vi "main.vi"() -> ()   [LabVIEW 2016]
uses:
  SALLV_Test/DataTypes/ackcmd.ctl
  SALLV_Test/DataTypes/logevent_arrays.ctl
  SALLV_Test/DataTypes/arrays.ctl
  SALLV_Test/DataTypes/logevent_scalars.ctl
  SALLV_Test/DataTypes/scalars.ctl
  SALLV_Test/VIs/Test_logEvent_summaryState.vi
  SALLV_Test/SALLV_Test.lvlib
panel:
  in  "TestID":u32
  out "Stop":bool
  in  "SummaryState":i32=5
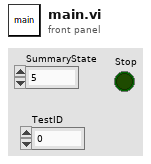
[diagram p1: front panel]
types:
  T1 = typedef "SALLV_Test.lvlib/ackcmd.ctl" = cluster{"cmdSeqNum":i32, "ack":i32, "error":i32, "result":string}
  T2 = typedef "SALLV_Test.lvlib/arrays.ctl" = cluster{"boolean0[5]":bool[], "byte0[5]":u8[], "char0":string, "short0[5]":i16[], "int0[5]":i32[], "long0[5]":i32[], "longLong0[5]":i64[], "octet0[5]":u8[], "unsignedShort0[5]":u16[], "unsignedInt0[5]":u32[], "unsignedLong0[5]":u32[], "float0[5]":sgl[], "double0[5]":dbl[]}
  T3 = typedef "SALLV_Test.lvlib/logevent_arrays.ctl" = cluster{"boolean0[5]":bool[], "byte0[5]":u8[], "char0":string, "short0[5]":i16[], "int0[5]":i32[], "long0[5]":i32[], "longLong0[5]":i64[], "octet0[5]":u8[], "unsignedShort0[5]":u16[], "unsignedInt0[5]":u32[], "unsignedLong0[5]":u32[], "float0[5]":sgl[], "double0[5]":dbl[], "priority":i32}
  T4 = typedef "SALLV_Test.lvlib/scalars.ctl" = cluster{"boolean0":bool, "byte0":u8, "char0":string, "short0":i16, "int0":i32, "long0":i32, "longLong0":i64, "octet0":u8, "unsignedShort0":u16, "unsignedInt0":u32, "unsignedLong0":u32, "float0":sgl, "double0":dbl, "string0":string}
  T5 = typedef "SALLV_Test.lvlib/logevent_scalars.ctl" = cluster{"boolean0":bool, "byte0":u8, "char0":string, "short0":i16, "int0":i32, "long0":i32, "longLong0":i64, "octet0":u8, "unsignedShort0":u16, "unsignedInt0":u32, "unsignedLong0":u32, "float0":sgl, "double0":dbl, "string0":string, "priority":i32}
  T6 = typedef "SALLV_Test.lvlib/command_setArrays.ctl" = cluster{"boolean0[5]":bool[], "byte0[5]":u8[], "char0":string, "short0[5]":i16[], "int0[5]":i32[], "long0[5]":i32[], "longLong0[5]":i64[], "octet0[5]":u8[], "unsignedShort0[5]":u16[], "unsignedInt0[5]":u32[], "unsignedLong0[5]":u32[], "float0[5]":sgl[], "double0[5]":dbl[]}
  T7 = typedef "SALLV_Test.lvlib/command_setScalars.ctl" = cluster{"boolean0":bool, "byte0":u8, "char0":string, "short0":i16, "int0":i32, "long0":i32, "longLong0":i64, "octet0":u8, "unsignedShort0":u16, "unsignedInt0":u32, "unsignedLong0":u32, "float0":sgl, "double0":dbl, "string0":string}
  T8 = typedef "SALLV_Test.lvlib/command_wait.ctl" = cluster{"cmdSeqNum":i32, "ack":i32, "duration":dbl}
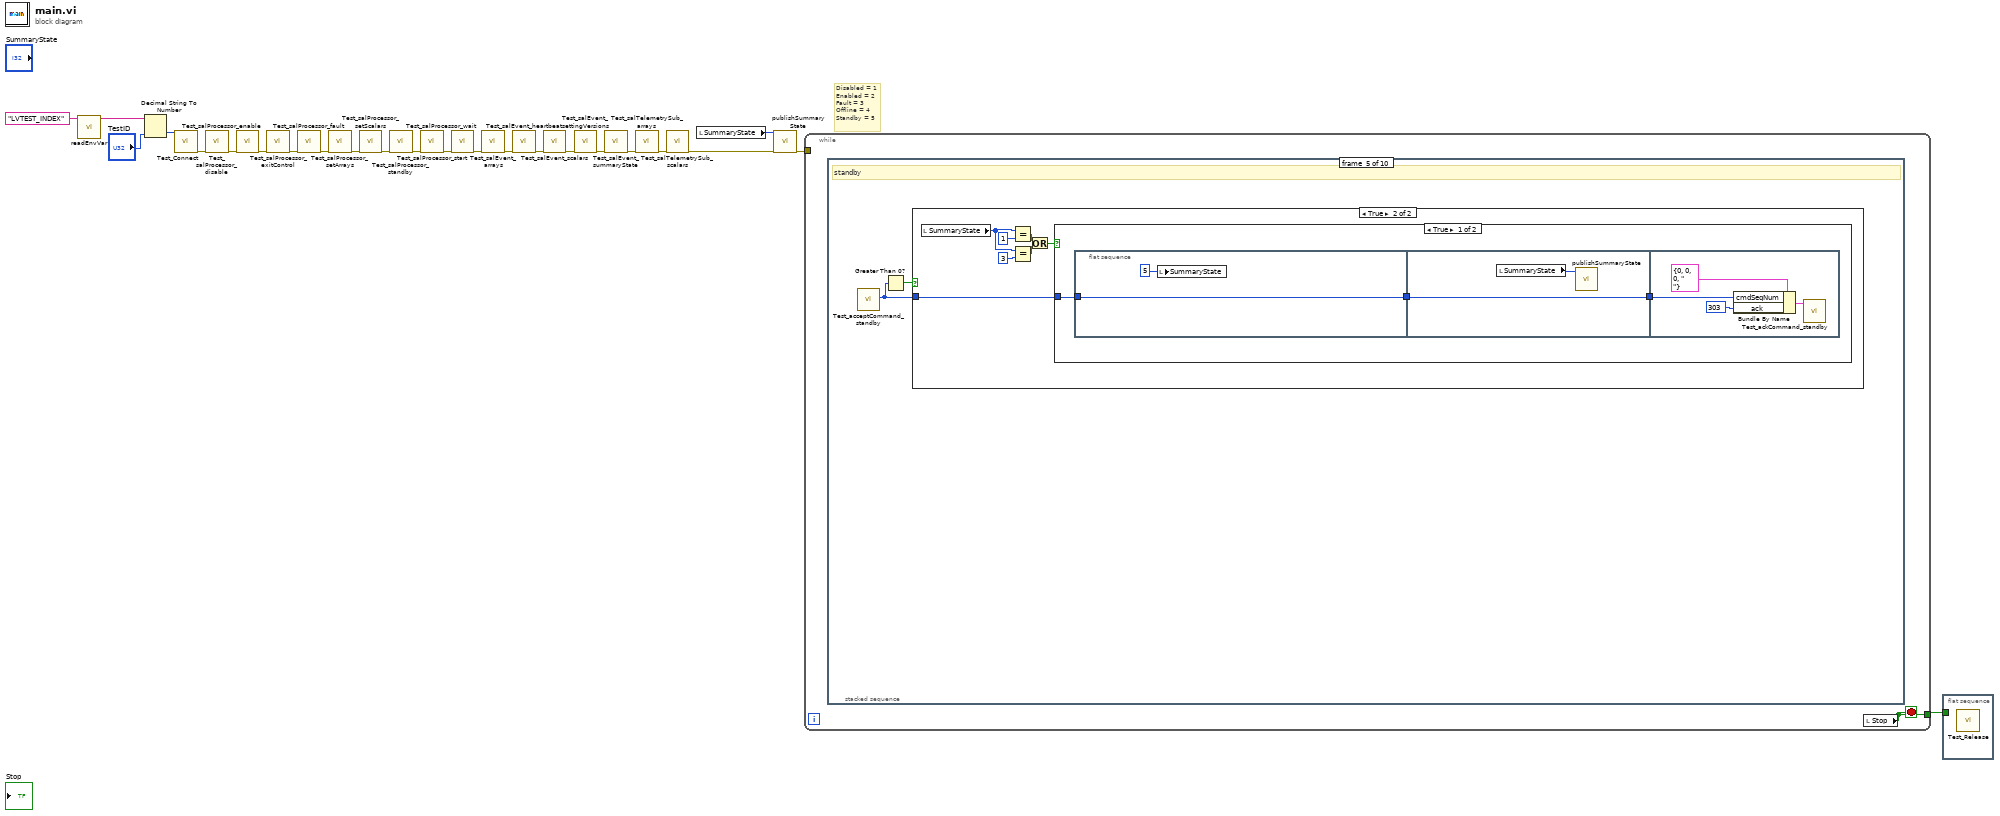
[diagram p0: block diagram]
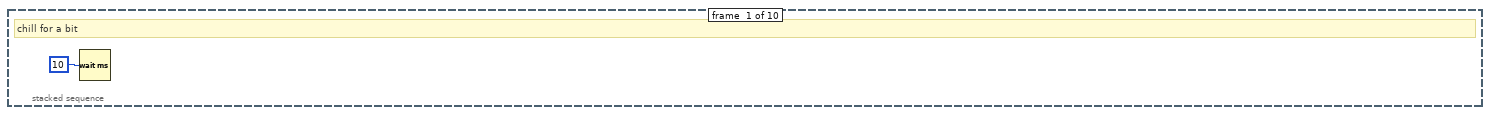
[diagram p2: hidden frame]
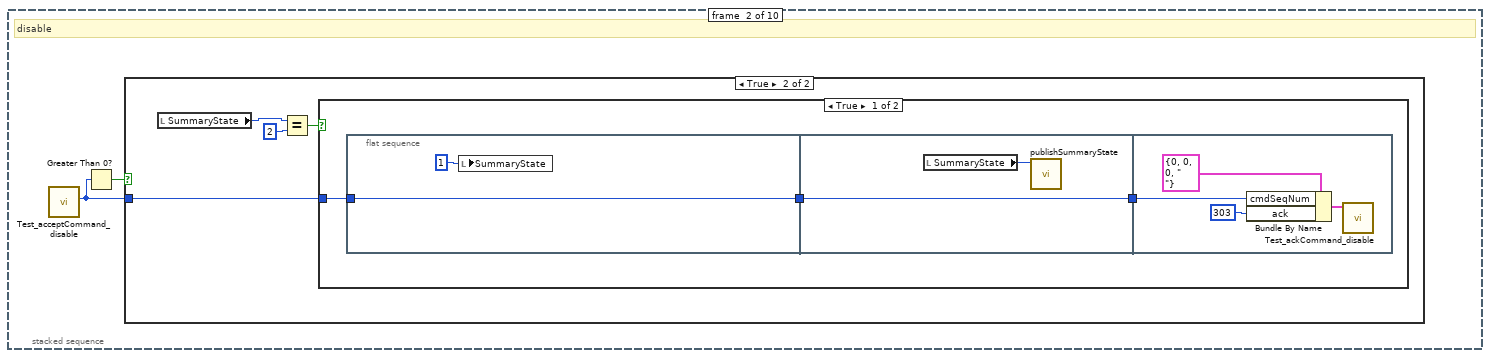
[diagram p3: hidden frame]
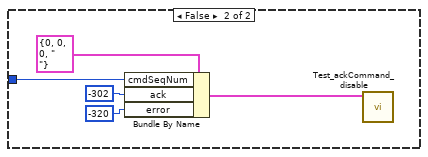
[diagram p5: hidden frame]
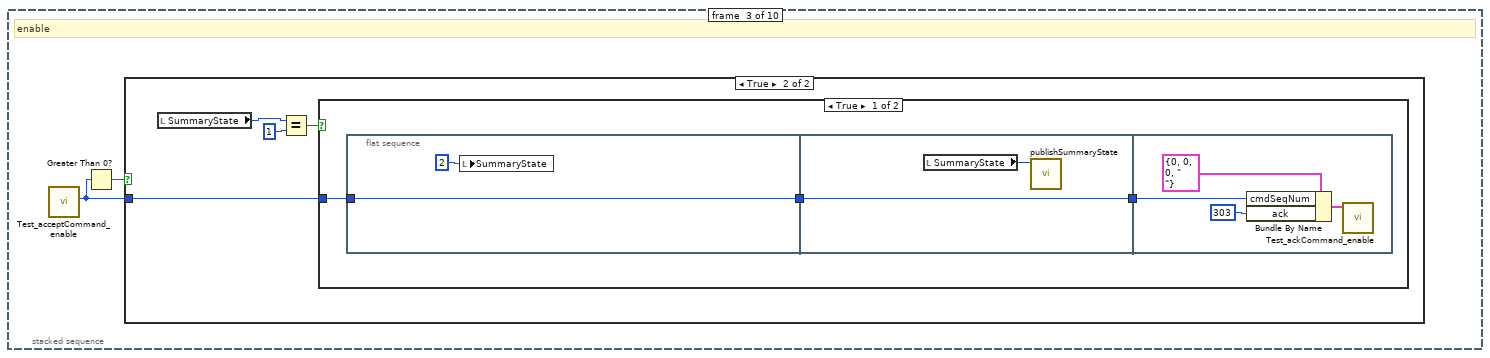
[diagram p6: hidden frame]
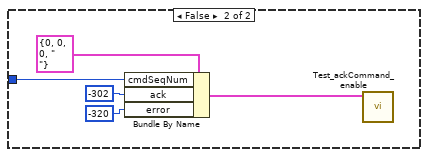
[diagram p8: hidden frame]
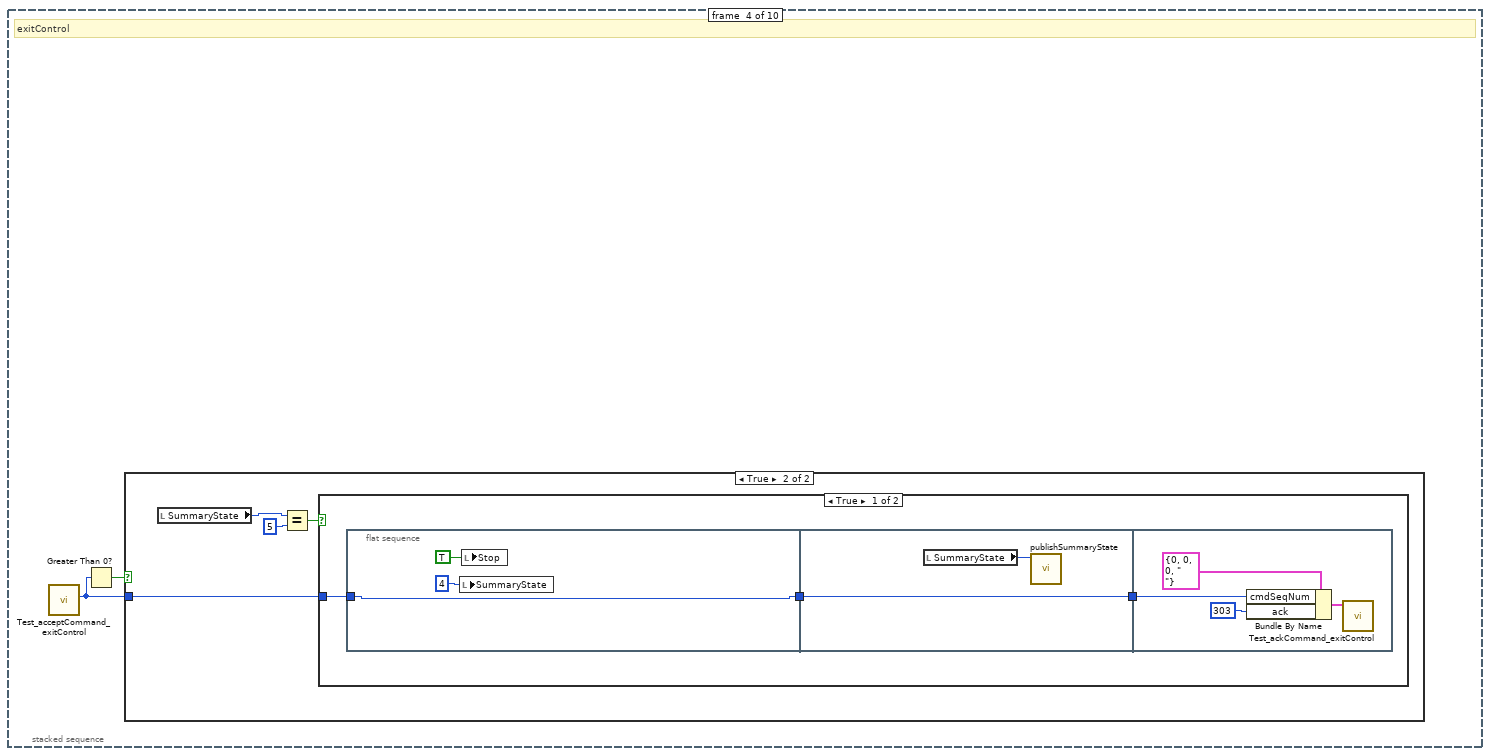
[diagram p9: hidden frame]
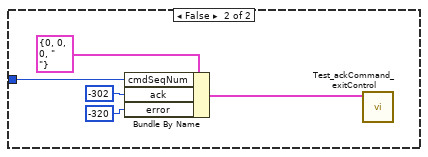
[diagram p11: hidden frame]
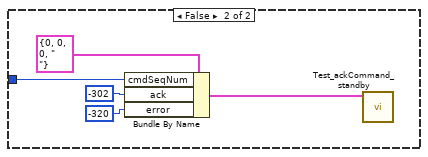
[diagram p13: hidden frame]
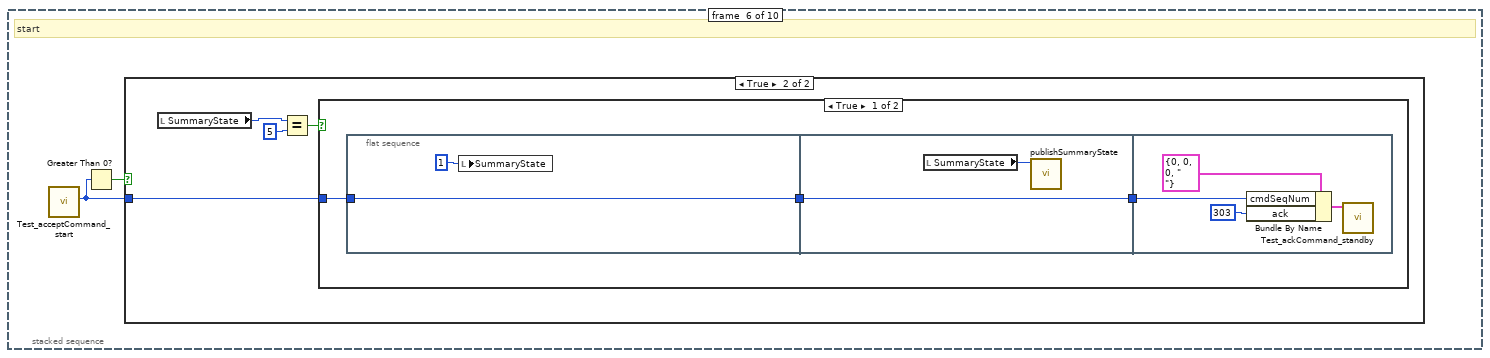
[diagram p14: hidden frame]
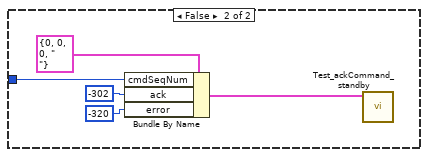
[diagram p16: hidden frame]
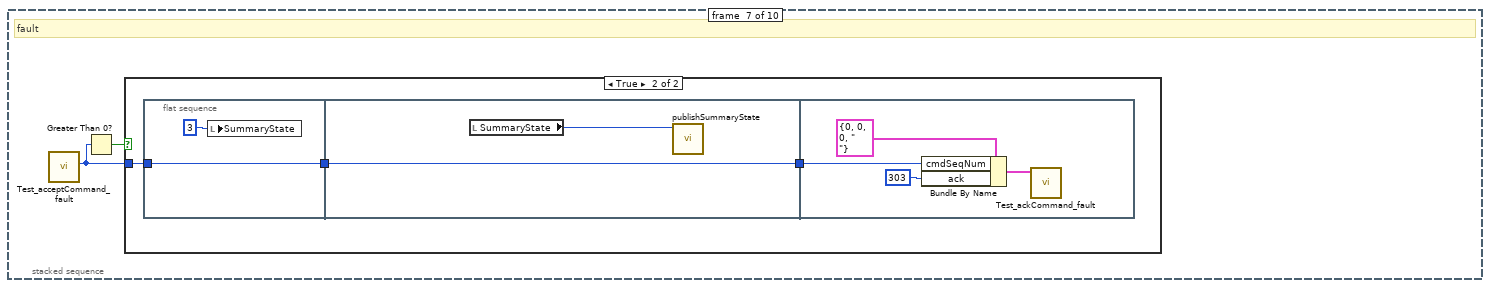
[diagram p17: hidden frame]
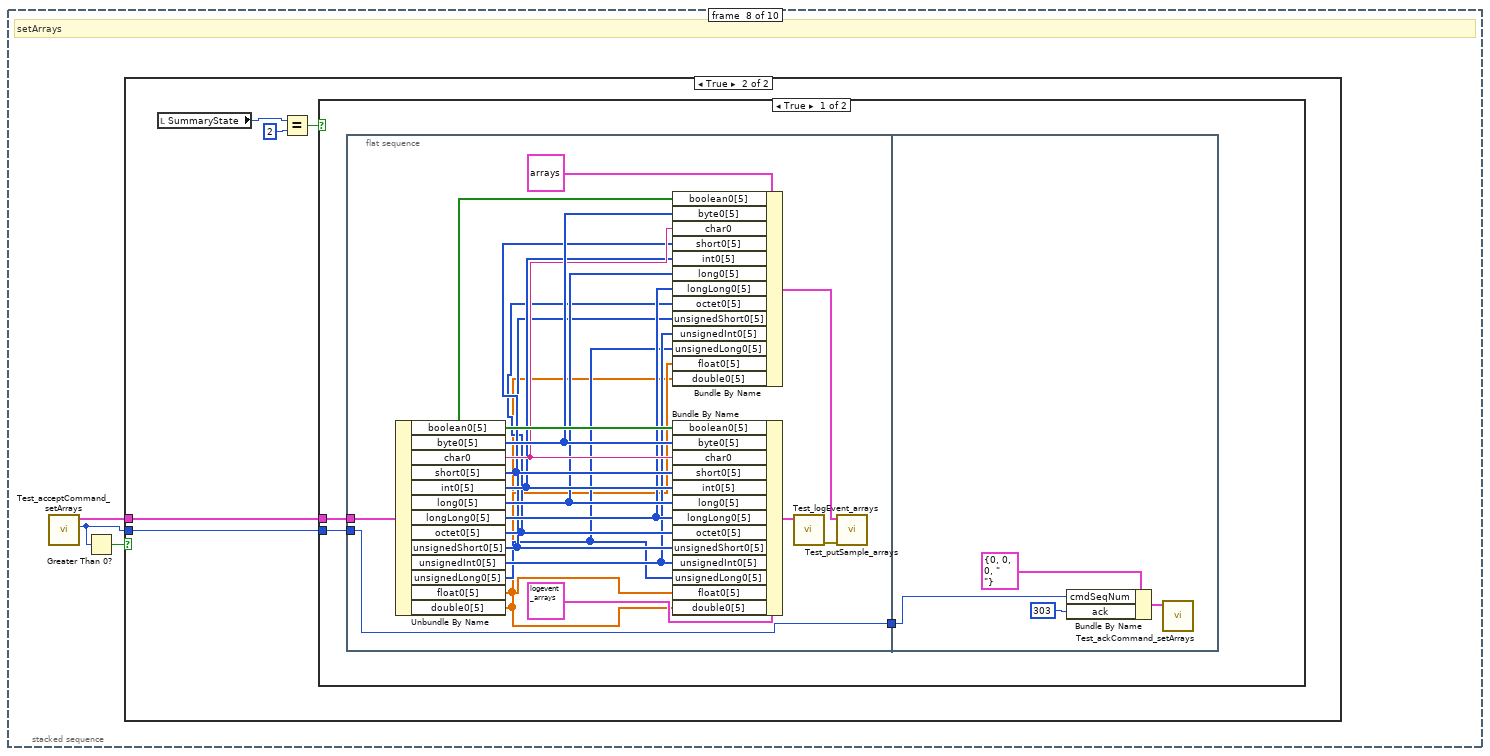
[diagram p19: hidden frame]
diagram:
  # "Disabled = 1\nEnabled = 2\nFault = 3\nOffline = 4\nStandby = 5"
  n1 = call "readEnvVar.vi"("command line"="LVTEST_INDEX") -> ("standard output"=w1:string)  [unwired: 10 in]
  n2 = Decimal String To Number(string=w1, default (0L)="TestID") -> (number=w3:u32)  [unwired: 1 in, 1 out]
  n3 = call "Test_Connect.vi"("TestID"=w3) -> ("error out"=w24:errorcluster)  [unwired: 9 in, 1 out]
  n4 = call "Test_salProcessor_disable.vi"("error in (no error)"=w24) -> ("error out"=w23:errorcluster)  [unwired: 9 in, 1 out]
  n5 = call "Test_salProcessor_enable.vi"("error in (no error)"=w23) -> ("error out"=w22:errorcluster)  [unwired: 9 in, 1 out]
  n6 = call "Test_salProcessor_exitControl.vi"("error in (no error)"=w22) -> ("error out"=w21:errorcluster)  [unwired: 9 in, 1 out]
  n7 = call "Test_salProcessor_fault.vi"("error in (no error)"=w21) -> ("error out"=w20:errorcluster)  [unwired: 9 in, 1 out]
  n8 = call "Test_salProcessor_setArrays.vi"("error in (no error)"=w20) -> ("error out"=w19:errorcluster)  [unwired: 9 in, 1 out]
  n9 = call "Test_salProcessor_setScalars.vi"("error in (no error)"=w19) -> ("error out"=w18:errorcluster)  [unwired: 9 in, 1 out]
  n10 = call "Test_salProcessor_standby.vi"("error in (no error)"=w18) -> ("error out"=w17:errorcluster)  [unwired: 9 in, 1 out]
  n11 = call "Test_salProcessor_start.vi"("error in (no error)"=w17) -> ("error out"=w16:errorcluster)  [unwired: 9 in, 1 out]
  n12 = call "Test_salProcessor_wait.vi"("error in (no error)"=w16) -> ("error out"=w15:errorcluster)  [unwired: 9 in, 1 out]
  n13 = call "Test_salEvent_arrays.vi"("error in (no error)"=w15) -> ("error out"=w14:errorcluster)  [unwired: 9 in, 1 out]
  n14 = call "Test_salEvent_heartbeat.vi"("error in (no error)"=w14) -> ("error out"=w13:errorcluster)  [unwired: 9 in, 1 out]
  n15 = call "Test_salEvent_scalars.vi"("error in (no error)"=w13) -> ("error out"=w12:errorcluster)  [unwired: 9 in, 1 out]
  n16 = call "Test_salEvent_settingVersions.vi"("error in (no error)"=w12) -> ("error out"=w11:errorcluster)  [unwired: 9 in, 1 out]
  n17 = call "Test_salEvent_summaryState.vi"("error in (no error)"=w11) -> ("error out"=w10:errorcluster)  [unwired: 9 in, 1 out]
  n18 = call "Test_salTelemetrySub_arrays.vi"("error in (no error)"=w10) -> ("error out"=w9:errorcluster)  [unwired: 9 in, 1 out]
  n19 = call "Test_salTelemetrySub_scalars.vi"("error in (no error)"=w9) -> ("error out"=w8:errorcluster)  [unwired: 9 in, 1 out]
  n20 = local read "SummaryState"() -> (w7:i32)
  n21 = call "publishSummaryState.vi"("error in (no error)"=w8, "SummaryState"=w7) -> ("error out"=w6:errorcluster)  [unwired: 9 in]
  n22 = while {
    tunnel: w6 -> [_]
    tunnel: [w25] -> w5
    stop <- w25 stop-if-true
    n23 = stacked-sequence {
      frame #0 {
        # "chill for a bit"
        n24 = Wait (ms)(milliseconds to wait=u32 10) -> ()  [unwired: 1 out]
      }
      frame #1 {
        # "disable"
        n25 = call "Test_acceptCommand_disable.vi"() -> ("function return"=w27:i32)  [unwired: 9 in, 2 out]
        n26 = Greater Than 0?(x=w27) -> (x > 0?=w28:bool)
        n27 = case shown="True" w28 {
          tunnel: w27 -> [_ w29]
          frame False {
          }
          frame True {
            n28 = local read "SummaryState"() -> (w32:i32)
            n29 = Equal?(x=w32, y=2) -> (x = y?=w30:bool)
            n30 = case shown="True" w30 {
              tunnel: w29 -> [w35 w48]
              frame True {
                n31 = flat-sequence {
                  tunnel: w35 -> [w37]
                  tunnel: [w37] -> w33
                  tunnel: [w39] -> w34
                  tunnel: w33 -> [w39]
                  tunnel: w34 -> [w40]
                  frame #0 {
                    n32 = local write "SummaryState"(1 ("SummaryState")) -> ()
                  }
                  frame #1 {
                    n33 = local read "SummaryState"() -> (w38:i32)
                    n34 = call "publishSummaryState.vi"("SummaryState"=w38) -> ()  [unwired: 10 in, 1 out]
                  }
                  frame #2 {
                    n35 = Bundle By Name(cluster=T1 {"cmdSeqNum"=0, "ack"=0, "error"=0, "result"="                                                                                                                                                                                                                                                                "} ("ackcmd_Ctl"), "cmdSeqNum"=w40, "ack"=303) -> (w41:T1)
                    n36 = call "Test_ackCommand_disable.vi"("ackcmd_Ctl"=w41) -> ()  [unwired: 8 in, 3 out]
                  }
                }
              }
              frame False {
                n37 = Bundle By Name(cluster=T1 {"cmdSeqNum"=0, "ack"=0, "error"=0, "result"="                                                                                                                                                                                                                                                                "} ("ackcmd_Ctl"), "cmdSeqNum"=w48, "ack"=-302, "error"=-320) -> (w45:T1)
                n38 = call "Test_ackCommand_disable.vi"("ackcmd_Ctl"=w45) -> ()  [unwired: 8 in, 3 out]
              }
            }
          }
        }
      }
      frame #2 {
        # "enable"
        n39 = call "Test_acceptCommand_enable.vi"() -> ("function return"=w49:i32)  [unwired: 9 in, 2 out]
        n40 = Greater Than 0?(x=w49) -> (x > 0?=w50:bool)
        n41 = case shown="True" w50 {
          tunnel: w49 -> [_ w51]
          frame False {
          }
          frame True {
            n42 = local read "SummaryState"() -> (w54:i32)
            n43 = Equal?(x=w54, y=1) -> (x = y?=w52:bool)
            n44 = case shown="True" w52 {
              tunnel: w51 -> [w57 w70]
              frame True {
                n45 = flat-sequence {
                  tunnel: w57 -> [w59]
                  tunnel: [w59] -> w55
                  tunnel: [w61] -> w56
                  tunnel: w55 -> [w61]
                  tunnel: w56 -> [w62]
                  frame #0 {
                    n46 = local write "SummaryState"(2 ("SummaryState")) -> ()
                  }
                  frame #1 {
                    n47 = local read "SummaryState"() -> (w60:i32)
                    n48 = call "publishSummaryState.vi"("SummaryState"=w60) -> ()  [unwired: 10 in, 1 out]
                  }
                  frame #2 {
                    n49 = Bundle By Name(cluster=T1 {"cmdSeqNum"=0, "ack"=0, "error"=0, "result"="                                                                                                                                                                                                                                                                "} ("ackcmd_Ctl"), "cmdSeqNum"=w62, "ack"=303) -> (w63:T1)
                    n50 = call "Test_ackCommand_enable.vi"("ackcmd_Ctl"=w63) -> ()  [unwired: 8 in, 3 out]
                  }
                }
              }
              frame False {
                n51 = Bundle By Name(cluster=T1 {"cmdSeqNum"=0, "ack"=0, "error"=0, "result"="                                                                                                                                                                                                                                                                "} ("ackcmd_Ctl"), "cmdSeqNum"=w70, "ack"=-302, "error"=-320) -> (w67:T1)
                n52 = call "Test_ackCommand_enable.vi"("ackcmd_Ctl"=w67) -> ()  [unwired: 8 in, 3 out]
              }
            }
          }
        }
      }
      frame #3 {
        # "exitControl"
        n53 = call "Test_acceptCommand_exitControl.vi"() -> ("function return"=w71:i32)  [unwired: 9 in, 2 out]
        n54 = Greater Than 0?(x=w71) -> (x > 0?=w72:bool)
        n55 = case shown="True" w72 {
          tunnel: w71 -> [_ w73]
          frame False {
          }
          frame True {
            n56 = local read "SummaryState"() -> (w76:i32)
            n57 = Equal?(x=w76, y=5) -> (x = y?=w74:bool)
            n58 = case shown="True" w74 {
              tunnel: w73 -> [w79 w93]
              frame True {
                n59 = flat-sequence {
                  tunnel: w79 -> [w82]
                  tunnel: [w82] -> w77
                  tunnel: [w84] -> w78
                  tunnel: w77 -> [w84]
                  tunnel: w78 -> [w85]
                  frame #0 {
                    n60 = local write "SummaryState"(4 ("SummaryState")) -> ()
                    n61 = local write "Stop"(TRUE ("Stop")) -> ()
                  }
                  frame #1 {
                    n62 = local read "SummaryState"() -> (w83:i32)
                    n63 = call "publishSummaryState.vi"("SummaryState"=w83) -> ()  [unwired: 10 in, 1 out]
                  }
                  frame #2 {
                    n64 = Bundle By Name(cluster=T1 {"cmdSeqNum"=0, "ack"=0, "error"=0, "result"="                                                                                                                                                                                                                                                                "} ("ackcmd_Ctl"), "cmdSeqNum"=w85, "ack"=303) -> (w86:T1)
                    n65 = call "Test_ackCommand_exitControl.vi"("ackcmd_Ctl"=w86) -> ()  [unwired: 8 in, 3 out]
                  }
                }
              }
              frame False {
                n66 = Bundle By Name(cluster=T1 {"cmdSeqNum"=0, "ack"=0, "error"=0, "result"="                                                                                                                                                                                                                                                                "} ("ackcmd_Ctl"), "cmdSeqNum"=w93, "ack"=-302, "error"=-320) -> (w90:T1)
                n67 = call "Test_ackCommand_exitControl.vi"("ackcmd_Ctl"=w90) -> ()  [unwired: 8 in, 3 out]
              }
            }
          }
        }
      }
      frame #4 {
        # "standby"
        n68 = call "Test_acceptCommand_standby.vi"() -> ("function return"=w94:i32)  [unwired: 9 in, 2 out]
        n69 = Greater Than 0?(x=w94) -> (x > 0?=w95:bool)
        n70 = case shown="True" w95 {
          tunnel: w94 -> [_ w101]
          frame False {
          }
          frame True {
            n71 = local read "SummaryState"() -> (w99:i32)
            n72 = Equal?(x=w99, y=1) -> (x = y?=w97:bool)
            n73 = Equal?(x=w99, y=3) -> (x = y?=w98:bool)
            n74 = Or(x=w97, y=w98) -> (x .or. y?=w96:bool)
            n75 = case shown="True" w96 {
              tunnel: w101 -> [w105 w118]
              frame True {
                n76 = flat-sequence {
                  tunnel: w105 -> [w107]
                  tunnel: [w107] -> w103
                  tunnel: [w109] -> w104
                  tunnel: w103 -> [w109]
                  tunnel: w104 -> [w110]
                  frame #0 {
                    n77 = local write "SummaryState"(5 ("SummaryState")) -> ()
                  }
                  frame #1 {
                    n78 = local read "SummaryState"() -> (w108:i32)
                    n79 = call "publishSummaryState.vi"("SummaryState"=w108) -> ()  [unwired: 10 in, 1 out]
                  }
                  frame #2 {
                    n80 = Bundle By Name(cluster=T1 {"cmdSeqNum"=0, "ack"=0, "error"=0, "result"="                                                                                                                                                                                                                                                                "} ("ackcmd_Ctl"), "cmdSeqNum"=w110, "ack"=303) -> (w111:T1)
                    n81 = call "Test_ackCommand_standby.vi"("ackcmd_Ctl"=w111) -> ()  [unwired: 8 in, 3 out]
                  }
                }
              }
              frame False {
                n82 = Bundle By Name(cluster=T1 {"cmdSeqNum"=0, "ack"=0, "error"=0, "result"="                                                                                                                                                                                                                                                                "} ("ackcmd_Ctl"), "cmdSeqNum"=w118, "ack"=-302, "error"=-320) -> (w115:T1)
                n83 = call "Test_ackCommand_standby.vi"("ackcmd_Ctl"=w115) -> ()  [unwired: 8 in, 3 out]
              }
            }
          }
        }
      }
      frame #5 {
        # "start"
        n84 = call "Test_acceptCommand_start.vi"() -> ("function return"=w119:i32)  [unwired: 9 in, 2 out]
        n85 = Greater Than 0?(x=w119) -> (x > 0?=w120:bool)
        n86 = case shown="True" w120 {
          tunnel: w119 -> [_ w121]
          frame False {
          }
          frame True {
            n87 = local read "SummaryState"() -> (w124:i32)
            n88 = Equal?(x=w124, y=5) -> (x = y?=w122:bool)
            n89 = case shown="True" w122 {
              tunnel: w121 -> [w127 w140]
              frame True {
                n90 = flat-sequence {
                  tunnel: w127 -> [w129]
                  tunnel: [w129] -> w125
                  tunnel: [w131] -> w126
                  tunnel: w125 -> [w131]
                  tunnel: w126 -> [w132]
                  frame #0 {
                    n91 = local write "SummaryState"(1 ("SummaryState")) -> ()
                  }
                  frame #1 {
                    n92 = local read "SummaryState"() -> (w130:i32)
                    n93 = call "publishSummaryState.vi"("SummaryState"=w130) -> ()  [unwired: 10 in, 1 out]
                  }
                  frame #2 {
                    n94 = Bundle By Name(cluster=T1 {"cmdSeqNum"=0, "ack"=0, "error"=0, "result"="                                                                                                                                                                                                                                                                "} ("ackcmd_Ctl"), "cmdSeqNum"=w132, "ack"=303) -> (w133:T1)
                    n95 = call "Test_ackCommand_standby.vi"("ackcmd_Ctl"=w133) -> ()  [unwired: 8 in, 3 out]
                  }
                }
              }
              frame False {
                n96 = Bundle By Name(cluster=T1 {"cmdSeqNum"=0, "ack"=0, "error"=0, "result"="                                                                                                                                                                                                                                                                "} ("ackcmd_Ctl"), "cmdSeqNum"=w140, "ack"=-302, "error"=-320) -> (w137:T1)
                n97 = call "Test_ackCommand_standby.vi"("ackcmd_Ctl"=w137) -> ()  [unwired: 8 in, 3 out]
              }
            }
          }
        }
      }
      frame #6 {
        # "fault"
        n98 = call "Test_acceptCommand_fault.vi"() -> ("function return"=w141:i32)  [unwired: 9 in, 2 out]
        n99 = Greater Than 0?(x=w141) -> (x > 0?=w142:bool)
        n100 = case shown="True" w142 {
          tunnel: w141 -> [_ w145]
          frame False {
          }
          frame True {
            n101 = flat-sequence {
              tunnel: w145 -> [w147]
              tunnel: [w147] -> w144
              tunnel: [w149] -> w143
              tunnel: w144 -> [w149]
              tunnel: w143 -> [w150]
              frame #0 {
                n102 = local write "SummaryState"(3 ("SummaryState")) -> ()
              }
              frame #1 {
                n103 = local read "SummaryState"() -> (w148:i32)
                n104 = call "publishSummaryState.vi"("SummaryState"=w148) -> ()  [unwired: 10 in, 1 out]
              }
              frame #2 {
                n105 = Bundle By Name(cluster=T1 {"cmdSeqNum"=0, "ack"=0, "error"=0, "result"="                                                                                                                                                                                                                                                                "} ("ackcmd_Ctl"), "cmdSeqNum"=w150, "ack"=303) -> (w151:T1)
                n106 = call "Test_ackCommand_fault.vi"("ackcmd_Ctl"=w151) -> ()  [unwired: 8 in, 3 out]
              }
            }
          }
        }
      }
      frame #7 {
        # "setArrays"
        n107 = call "Test_acceptCommand_setArrays.vi"() -> ("function return"=w155:i32, "command_setArrays_Ctl out"=w154:T6)  [unwired: 9 in, 1 out]
        n108 = Greater Than 0?(x=w155) -> (x > 0?=w156:bool)
        n109 = case shown="True" w156 {
          tunnel: w155 -> [_ w158]
          tunnel: w154 -> [_ w157]
          frame False {
          }
          frame True {
            n110 = local read "SummaryState"() -> (w161:i32)
            n111 = Equal?(x=w161, y=2) -> (x = y?=w159:bool)
            n112 = case shown="True" w159 {
              tunnel: w158 -> [w164 w193]
              tunnel: w157 -> [w163 _]
              frame True {
                n113 = flat-sequence {
                  tunnel: w164 -> [w184]
                  tunnel: [w184] -> w162
                  tunnel: w163 -> [w183]
                  tunnel: w162 -> [w185]
                  frame #0 {
                    n114 = Unbundle By Name(w183) -> ("boolean0[5]"=w180:bool[], "byte0[5]"=w179:u8[], "char0"=w178:string, "short0[5]"=w177:i16[], "int0[5]"=w176:i32[], "long0[5]"=w175:i32[], "longLong0[5]"=w174:i64[], "octet0[5]"=w173:u8[], "unsignedShort0[5]"=w172:u16[], "unsignedInt0[5]"=w171:u32[], "unsignedLong0[5]"=w170:u32[], "float0[5]"=w169:sgl[], "double0[5]"=w168:dbl[])
                    n115 = Bundle By Name(cluster=T2 {"boolean0[5]"=[FALSE, FALSE, FALSE, FALSE, FALSE], "byte0[5]"=[0, 0, 0, 0, 0], "char0"="", "short0[5]"=[0, 0, 0, 0, 0], "int0[5]"=[0, 0, 0, 0, 0], "long0[5]"=[0, 0, 0, 0, 0], "longLong0[5]"=[0, 0, 0, 0, 0], "octet0[5]"=[0, 0, 0, 0, 0], "unsignedShort0[5]"=[0, 0, 0, 0, 0], "unsignedInt0[5]"=[0, 0, 0, 0, 0], "unsignedLong0[5]"=[0, 0, 0, 0, 0], "float0[5]"=[0.0, 0.0, 0.0, 0.0, 0.0], "double0[5]"=[0.0, 0.0, 0.0, 0.0, 0.0]} ("arrays"), "boolean0[5]"=w180, "byte0[5]"=w179, "char0"=w178, "short0[5]"=w177, "int0[5]"=w176, "long0[5]"=w175, "longLong0[5]"=w174, "octet0[5]"=w173, "unsignedShort0[5]"=w172, "unsignedInt0[5]"=w171, "unsignedLong0[5]"=w170, "float0[5]"=w169, "double0[5]"=w168) -> (w167:T2)
                    n116 = Bundle By Name(cluster=T3 {"boolean0[5]"=[FALSE, FALSE, FALSE, FALSE, FALSE], "byte0[5]"=[0, 0, 0, 0, 0], "char0"="", "short0[5]"=[0, 0, 0, 0, 0], "int0[5]"=[0, 0, 0, 0, 0], "long0[5]"=[0, 0, 0, 0, 0], "longLong0[5]"=[0, 0, 0, 0, 0], "octet0[5]"=[0, 0, 0, 0, 0], "unsignedShort0[5]"=[0, 0, 0, 0, 0], "unsignedInt0[5]"=[0, 0, 0, 0, 0], "unsignedLong0[5]"=[0, 0, 0, 0, 0], "float0[5]"=[0.0, 0.0, 0.0, 0.0, 0.0], "double0[5]"=[0.0, 0.0, 0.0, 0.0, 0.0], "priority"=0} ("logevent_arrays"), "boolean0[5]"=w180, "byte0[5]"=w179, "char0"=w178, "short0[5]"=w177, "int0[5]"=w176, "long0[5]"=w175, "longLong0[5]"=w174, "octet0[5]"=w173, "unsignedShort0[5]"=w172, "unsignedInt0[5]"=w171, "unsignedLong0[5]"=w170, "float0[5]"=w169, "double0[5]"=w168) -> (w166:T3)
                    n117 = call "Test_logEvent_arrays.vi"("logevent_arrays_Ctl"=w166) -> ("error out"=w165:errorcluster)  [unwired: 8 in, 2 out]
                    n118 = call "Test_putSample_arrays.vi"("error in (no error)"=w165, "arrays_Ctl"=w167) -> ()  [unwired: 7 in, 3 out]
                  }
                  frame #1 {
                    n119 = Bundle By Name(cluster=T1 {"cmdSeqNum"=0, "ack"=0, "error"=0, "result"="                                                                                                                                                                                                                                                                "} ("ackcmd_Ctl"), "cmdSeqNum"=w185, "ack"=303) -> (w186:T1)
                    n120 = call "Test_ackCommand_setArrays.vi"("ackcmd_Ctl"=w186) -> ()  [unwired: 8 in, 3 out]
                  }
                }
              }
              frame False {
                n121 = Bundle By Name(cluster=T1 {"cmdSeqNum"=0, "ack"=0, "error"=0, "result"="                                                                                                                                                                                                                                                                "} ("ackcmd_Ctl"), "cmdSeqNum"=w193, "ack"=-302, "error"=-320) -> (w190:T1)
                n122 = call "Test_ackCommand_setArrays.vi"("ackcmd_Ctl"=w190) -> ()  [unwired: 8 in, 3 out]
              }
            }
          }
        }
      }
      frame #8 {
        # "setScalars"
        n123 = call "Test_acceptCommand_setScalars.vi"() -> ("function return"=w195:i32, "command_setScalars_Ctl out"=w194:T7)  [unwired: 9 in, 1 out]
        n124 = Greater Than 0?(x=w195) -> (x > 0?=w196:bool)
        n125 = case shown="True" w196 {
          tunnel: w195 -> [_ w198]
          tunnel: w194 -> [_ w197]
          frame False {
          }
          frame True {
            n126 = local read "SummaryState"() -> (w201:i32)
            n127 = Equal?(x=w201, y=2) -> (x = y?=w199:bool)
            n128 = case shown="True" w199 {
              tunnel: w198 -> [w204 w234]
              tunnel: w197 -> [w203 _]
              frame True {
                n129 = flat-sequence {
                  tunnel: w204 -> [w225]
                  tunnel: [w225] -> w202
                  tunnel: w203 -> [w224]
                  tunnel: w202 -> [w226]
                  frame #0 {
                    n130 = Unbundle By Name(w224) -> ("boolean0"=w221:bool, "byte0"=w220:u8, "char0"=w219:string, "short0"=w218:i16, "int0"=w217:i32, "long0"=w216:i32, "longLong0"=w215:i64, "octet0"=w214:u8, "unsignedShort0"=w213:u16, "unsignedInt0"=w212:u32, "unsignedLong0"=w211:u32, "float0"=w210:sgl, "double0"=w209:dbl, "string0"=w206:string)
                    n131 = Bundle By Name(cluster=T4 {"boolean0"=FALSE, "byte0"=0, "char0"="", "short0"=0, "int0"=0, "long0"=0, "longLong0"=0, "octet0"=0, "unsignedShort0"=0, "unsignedInt0"=0, "unsignedLong0"=0, "float0"=0.0, "double0"=0.0, "string0"="                    "} ("scalars"), "boolean0"=w221, "byte0"=w220, "char0"=w219, "short0"=w218, "int0"=w217, "long0"=w216, "longLong0"=w215, "octet0"=w214, "unsignedShort0"=w213, "unsignedInt0"=w212, "unsignedLong0"=w211, "float0"=w210, "double0"=w209, "string0"=w206) -> (w208:T4)
                    n132 = Bundle By Name(cluster=T5 {"boolean0"=FALSE, "byte0"=0, "char0"="", "short0"=0, "int0"=0, "long0"=0, "longLong0"=0, "octet0"=0, "unsignedShort0"=0, "unsignedInt0"=0, "unsignedLong0"=0, "float0"=0.0, "double0"=0.0, "string0"="                    ", "priority"=0} ("logevent_scalars"), "boolean0"=w221, "byte0"=w220, "char0"=w219, "short0"=w218, "int0"=w217, "long0"=w216, "longLong0"=w215, "octet0"=w214, "unsignedShort0"=w213, "unsignedInt0"=w212, "unsignedLong0"=w211, "float0"=w210, "double0"=w209, "string0"=w206) -> (w205:T5)
                    n133 = call "Test_logEvent_scalars.vi"("logevent_scalars_Ctl"=w205) -> ("error out"=w207:errorcluster)  [unwired: 8 in, 2 out]
                    n134 = call "Test_putSample_scalars.vi"("error in (no error)"=w207, "scalars_Ctl"=w208) -> ()  [unwired: 7 in, 3 out]
                  }
                  frame #1 {
                    n135 = Bundle By Name(cluster=T1 {"cmdSeqNum"=0, "ack"=0, "error"=0, "result"="                                                                                                                                                                                                                                                                "} ("ackcmd_Ctl"), "cmdSeqNum"=w226, "ack"=303) -> (w227:T1)
                    n136 = call "Test_ackCommand_setScalars.vi"("ackcmd_Ctl"=w227) -> ()  [unwired: 8 in, 3 out]
                  }
                }
              }
              frame False {
                n137 = Bundle By Name(cluster=T1 {"cmdSeqNum"=0, "ack"=0, "error"=0, "result"="                                                                                                                                                                                                                                                                "} ("ackcmd_Ctl"), "cmdSeqNum"=w234, "ack"=-302, "error"=-320) -> (w231:T1)
                n138 = call "Test_ackCommand_setScalars.vi"("ackcmd_Ctl"=w231) -> ()  [unwired: 8 in, 3 out]
              }
            }
          }
        }
      }
      frame #9 {
        # "wait"
        n139 = call "Test_acceptCommand_wait.vi"() -> ("function return"=w236:i32, "command_wait_Ctl out"=w235:T8)  [unwired: 9 in, 1 out]
        n140 = Greater Than 0?(x=w236) -> (x > 0?=w237:bool)
        n141 = case shown="True" w237 {
          tunnel: w236 -> [_ w239]
          tunnel: w235 -> [_ w238]
          frame False {
          }
          frame True {
            n142 = local read "SummaryState"() -> (w242:i32)
            n143 = Equal?(x=w242, y=2) -> (x = y?=w240:bool)
            n144 = case shown="True" w240 {
              tunnel: w239 -> [w245 w260]
              tunnel: w238 -> [w244 _]
              frame True {
                n145 = flat-sequence {
                  tunnel: w245 -> [w251]
                  tunnel: [w251] -> w243
                  tunnel: w244 -> [w250]
                  tunnel: w243 -> [w252]
                  frame #0 {
                    n146 = Unbundle By Name(w250) -> ("duration"=w249:dbl)
                    n147 = Multiply(x=w249, y=1000.0) -> (x*y=w247:dbl)
                    n148 = To Unsigned Long Integer(number=w247) -> (unsigned 32bit integer=w246:u32)
                    n149 = Wait (ms)(milliseconds to wait=w246) -> ()  [unwired: 1 out]
                  }
                  frame #1 {
                    n150 = Bundle By Name(cluster=T1 {"cmdSeqNum"=0, "ack"=0, "error"=0, "result"="                                                                                                                                                                                                                                                                "} ("ackcmd_Ctl"), "cmdSeqNum"=w252, "ack"=303) -> (w253:T1)
                    n151 = call "Test_ackCommand_wait.vi"("ackcmd_Ctl"=w253) -> ()  [unwired: 8 in, 3 out]
                  }
                }
              }
              frame False {
                n152 = Bundle By Name(cluster=T1 {"cmdSeqNum"=0, "ack"=0, "error"=0, "result"="                                                                                                                                                                                                                                                                "} ("ackcmd_Ctl"), "cmdSeqNum"=w260, "ack"=-302, "error"=-320) -> (w257:T1)
                n153 = call "Test_ackCommand_wait.vi"("ackcmd_Ctl"=w257) -> ()  [unwired: 8 in, 3 out]
              }
            }
          }
        }
      }
    }
    n154 = local read "Stop"() -> (w25:bool)
  }
  n155 = flat-sequence {
    tunnel: w5 -> [_]
    frame #0 {
      n156 = call "Test_Release.vi"() -> ()  [unwired: 10 in, 2 out]
    }
  }
